vi "TEB Global.vi"() -> ()   [LabVIEW 2010]
panel:
  in  "Post processing list":string[](array[string])
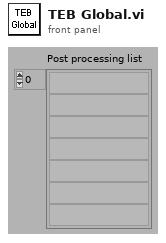
[diagram p1: front panel]
diagram:
